vi "editScriptEvent.vi"(6 "delayAll":bool=TRUE, 7 "selectedIndex":i32, 8 "error in (no error)":errorcluster, 9 "index":i32=-1, 10 "ScriptEvent":refnum<class "ScriptEvent.lvclass">, 11 "ScriptEventList in":refnum<class "ScriptEventList.lvclass">) -> (0 "error out":errorcluster, 3 "ScriptEventList out":refnum<class "ScriptEventList.lvclass">)   [LabVIEW 2011, in "Tools.lvlib" / "Scripting.lvlib" / "ScriptEventList.lvclass"]
uses:
  ScriptEventList.lvclass
  ScriptEvent.lvclass
  ScriptEventList.lvclass/ScriptEventList.ctl
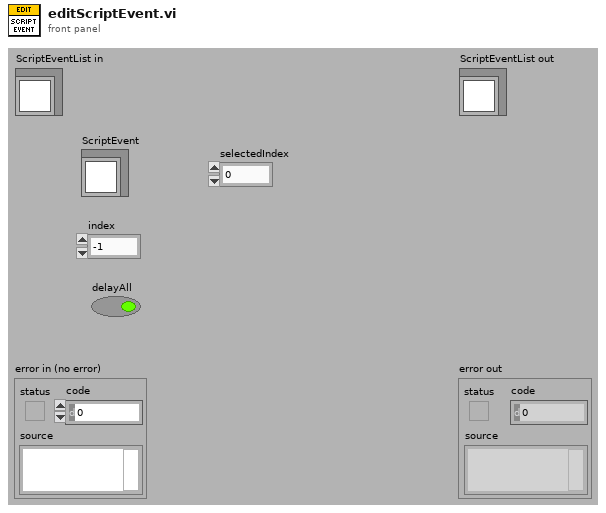
[diagram p1: front panel]
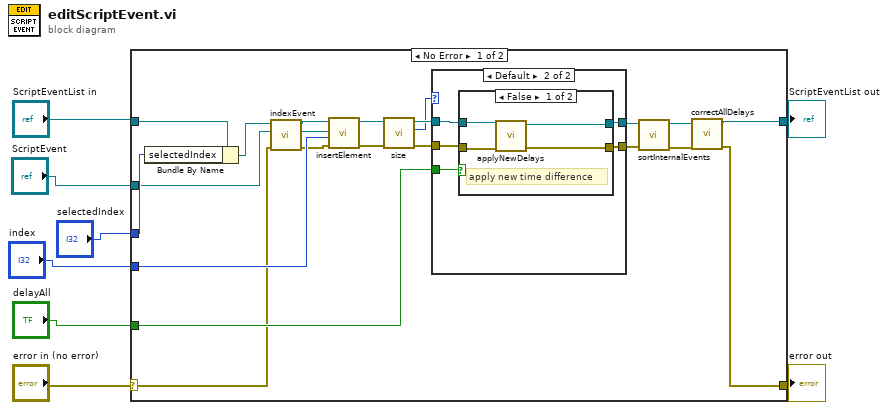
[diagram p0: block diagram]
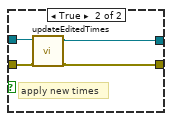
[diagram p3: hidden frame]
diagram:
  n1 = case shown="No Error" "error in (no error)" {
    selector: "error in (no error)" -> [w23 w46]
    tunnel: [w9 w46] -> w1
    tunnel: [w10 w45] -> w2
    tunnel: "ScriptEventList in" -> [w28 w45]
    tunnel: "ScriptEvent" -> [w25 _]
    tunnel: "delayAll" -> [w29 _]
    tunnel: "index" -> [w26 _]
    tunnel: "selectedIndex" -> [w27 _]
    frame No Error {
      n2 = Bundle By Name(cluster=w28, "selectedIndex"=w27) -> (w20:refnum<class "ScriptEventList.lvclass">)
      n3 = call "indexEvent.vi"("error in (no error)"=w23, "ScriptEvent"=w25, "ScriptEventList in"=w20) -> ("error out"=w24:errorcluster, "ScriptEvent out"=w22:refnum<class "ScriptEvent.lvclass">, "ScriptEventList out"=w21:refnum<class "ScriptEventList.lvclass">)  [unwired: 5 in, 1 out]
      n4 = call "insertElement.vi"("error in (no error)"=w24, "index"=w26, "ScriptEvent"=w22, "ScriptEventList in"=w21) -> ("error out"=w17:errorcluster, "ScriptEventList out"=w18:refnum<class "ScriptEventList.lvclass">)  [unwired: 6 in]
      n5 = call "size.vi"("error in (no error)"=w17, "ScriptEventList in"=w18) -> ("error out"=w16:errorcluster, "size"=w15:i32, "ScriptEventList out"=w19:refnum<class "ScriptEventList.lvclass">)  [unwired: 7 in]
      n6 = case shown="Default" w15 {
        tunnel: w29 -> [_ w36]
        tunnel: [w31 w35] -> w14
        tunnel: [w30 w34] -> w13
        tunnel: w19 -> [w31 w33]
        tunnel: w16 -> [w30 w32]
        frame 1 {
        }
        frame Default {
          n7 = case shown="False" w36 {
            tunnel: w33 -> [w40 w44]
            tunnel: w32 -> [w39 w42]
            tunnel: [w38 w43] -> w35
            tunnel: [w37 w41] -> w34
            frame False {
              # "apply new time difference"
              n8 = call "applyNewDelays.vi"("error in (no error)"=w39, "ScriptEventList in"=w40) -> ("error out"=w37:errorcluster, "ScriptEventList out"=w38:refnum<class "ScriptEventList.lvclass">)  [unwired: 8 in]
            }
            frame True {
              # "apply new times"
              n9 = call "updateEditedTimes.vi"("error in (no error)"=w42, "ScriptEventList in"=w44) -> ("error out"=w41:errorcluster, "ScriptEventList out"=w43:refnum<class "ScriptEventList.lvclass">)  [unwired: 8 in]
            }
          }
        }
      }
      n10 = call "sortInternalEvents.vi"("error in (no error)"=w13, "ScriptEventList in"=w14) -> ("error out"=w11:errorcluster, "ScriptEventList out"=w12:refnum<class "ScriptEventList.lvclass">)  [unwired: 8 in]
      n11 = call "correctAllDelays.vi"("error in (no error)"=w11, "ScriptEventList in"=w12) -> ("error out"=w9:errorcluster, "ScriptEventList out"=w10:refnum<class "ScriptEventList.lvclass">)  [unwired: 8 in]
    }
    frame Error {
    }
  }
  "error out" <- w1
  "ScriptEventList out" <- w2
